vi "Load Kernel.vi"(8 "Error In":errorcluster, 9 "Kernel Name":string, 10 "Program Handle":T1, 11 "Device In":T2) -> (0 "Error Out":errorcluster, 1 "Kernel Handle":T3, 2 "Program Handle out":T1, 3 "Device Out":T2)   [LabVIEW 2012]
doc: "Loads a kernel from a program."
uses:
  Non-User VIs/Controls/Kernel Handle.ctl
  Non-User VIs/Controls/Device ID.ctl
  Non-User VIs/Controls/Program Handle.ctl
  Non-User VIs/Error Checking/Add Error Functional Global.vi
  OpenCLV x64.lvlib
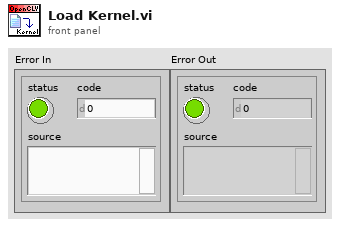
[diagram p1: front panel]
types:
  T1 = typedef "OpenCLV x64.lvlib/Program Handle.ctl" = u64
  T2 = typedef "OpenCLV x64.lvlib/Device ID.ctl" = u64
  T3 = typedef "OpenCLV x64.lvlib/Kernel Handle.ctl" = u64
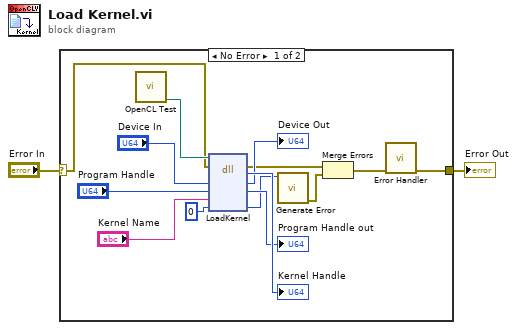
[diagram p0: block diagram]
diagram:
  n1 = case shown="No Error" "Error In" {
    selector: "Error In" -> [w3 w17]
    tunnel: [w7 w17] -> w1
    frame No Error {
      n2 = call "OpenCL Test.vi"() -> ("DLL To Use"=w8:path)  [unwired: 11 in]
      n3 = dll-call lib="C:/Users/bme-amcelroy-la/Desktop/OpenCLV/trunk/OpenCLV_x64_1.0/OpenCLV_x64.dll" fn="LoadKernel"(path in=w8, error in=w3, "Device In"="Device In", "Program"="Program Handle", "Kernel Name"="Kernel Name", "Error"=0) -> (error out=w5:errorcluster, "Kernel Handle"=→"Kernel Handle":u64, "Device In"=→"Device Out":u64, "Program"=→"Program Handle out":u64, "Error"=w10:i32)  [unwired: 2 in, 1 out]
      n4 = call "Generate Error.vi"("Error"=w10) -> ("error out"=w6:errorcluster)  [unwired: 10 in]
      n5 = Merge Errors(w5, w6) -> (w4:errorcluster)
      n6 = call-poly "Error Handler.vi"("Error In"=w4) -> ("Error Out"=w7:errorcluster)  [unwired: 10 in]
    }
    frame Error {
    }
  }
  "Error Out" <- w1
